vi "Process.vi"(8 "error in":errorcluster, 11 "DAQ_Manager":refnum<class "DAQ_Manager.lvclass">) -> (0 "error out":errorcluster, 3 "DAQ_Manager out":refnum<class "DAQ_Manager.lvclass">)   [LabVIEW 2016, in "DAQ_Manager.lvclass"]
doc: "---------------------------------------------------------------\nJKI State Machine Objects™\nhttp://jki.net/state-machine-objects/\nCopyright (C) 2005-2015, JKI <info@jki.net>\nALL RIGHTS RESERVED"
uses:
  DAQ_Manager.lvclass
  C:/Program Files (x86)/National Instruments/LabVIEW 2016/vi.lib/JKI/JKI SMO/SMO/SMO.lvclass
  DAQ/Typedefs/DAQ_Config.ctl
  DAQ/Typedefs/PrivateEvents--DAQ.AI.Channels.ctl
  DAQ/Typedefs/DAQ_Type.ctl
  DAQ/Typedefs/DAQ_SamplingInfo.ctl
  DAQ/Typedefs/DAQ_SamplingMode.ctl
  DAQmx.AI/Typedefs/DAQmx.AI_Config.ctl
  DAQmx.AI/Typedefs/AI.Coupling-enum.ctl
  DAQmx.AI/Typedefs/AI.Terminal-enum.ctl
  DAQmx.AO/Typedefs/DAQmx.AO_Config.ctl
  DAQmx.AO/Typedefs/AO.Terminal-enum.ctl
  <vilib>/JKI/JKI SMO/SMO/Typedefs/SMOState --Enum.ctl
  <vilib>/JKI/JKI SMO/SMO/Typedefs/Parent Call--Enum.ctl
  Typedefs/PrivateEvents--DAQ_Manager.setDAQConfig.ctl
  DAQ/Typedefs/PublicEvents--DAQ.Read.ctl
  DAQ/Typedefs/PublicEvents--DAQ.Write.ctl
  DAQ_Manager.lvclass/DAQ_Manager.ctl
  DAQ/DAQ.lvclass
  DAQmx/DAQmx.lvclass
  C:/user/patrick/hg/levy_inst_lockin.SMO/lvsrc/SMOs/DAQ/DAQ.lvclass
  DAQmx.AI/DAQmx.AI.lvclass
  C:/user/patrick/hg/levy_inst_lockin.SMO/lvsrc/SMOs/DAQmx/DAQmx.lvclass
  DAQmx.AO/DAQmx.AO.lvclass
  <vilib>/JKI/JKI SMO/SMO/SMO.lvclass
panel:
  out "Array":T1[](array[typedef])
  in  "Update Config?":bool
  in  "DAQmx.AO.config":T2[](array[typedef])=[{"output terminal configuration"=-1}] {"output terminal configuration" items=["Default"=-1, "RSE"=10083, "Differential"=10106, "Pseudodifferential"=12529]}
  in  "DAQmx.AI.config":T4[](array[typedef])=[{"AI.Coupling"=10045, "input terminal configuration "=-1}] {"input terminal configuration" items=["default"=-1, "RSE"=10083, "NRSE"=10078, "Differential"=10106, "Pseudodifferential"=12529]; "AI.Coupling" items=["AC"=10045, "DC"=10050, "GND"=10066]}
  in  "DAQ.Config (AO)":T7[](array[typedef])=[{"Channels"="PXI1Slot2/ao0", "DAQ_Type"=enum."AO", "minimum value"=-10.0, "maximum value"=10.0, "DAQ_SamplingInfo"={"Fs"=1000.0, "#s"=1000}, "DAQ_SamplingMode"=enum."Continuous"}] {"maximum value" format="%0.2f"; "minimum value" format="%0.2f"}
  in  "DAQ.Config (AI)":T7[](array[typedef])=[{"Channels"="PXI1Slot2/ai0", "DAQ_Type"=enum."AI", "minimum value"=-10.0, "maximum value"=10.0, "DAQ_SamplingInfo"={"Fs"=1000.0, "#s"=1000}, "DAQ_SamplingMode"=enum."Continuous"}] {"maximum value" format="%0.2f"; "minimum value" format="%0.2f"}
  in  "DAQmx Physical Channels (AO)":tag="PXI1Slot2/ao0:1, PXI1Slot3/ao0:1, PXI1Slot4/ao0:1, PXI1Slot5/ao0:1"
  in  "DAQmx Physical Channels (AI)":tag="PXI1Slot2/ai0:1, PXI1Slot3/ai0:1, PXI1Slot4/ai0:1, PXI1Slot5/ai0:1"
  in  "Simulate?":bool
  # "1. Make a lot of these controls hidden on default Main UI\n    (eg, output terminal)\n2. DAQ.Config etc should be arrays, with each element per device\n3. Make use of most recent lockin controls on front panel\n-- use new enums and arrays per channel/device\n4. DAQ_Manager needs an API for setting the DAQ config (setConfig?)\n5. In process.vi if any Config settings are changed: go to:\nDAQ: stop SMO\nDAQ: init\nDAQ: start SMO\n6. I don't think these need to be controls here in process.vi, they can just be\nchanged through public methods."
  # "DAQ Manager Process.vi"
  # "For instructions on how to use the JKI State Machine Objects, examples and video tutorials, visit:\nhttp://jki.net/state-machine-objects/\n\nJKI State Machine Objects™\nhttp://jki.net/state-machine-objects/\nCopyright (C) 2005-2015, JKI <info@jki.net>\nALL RIGHTS RESERVED"
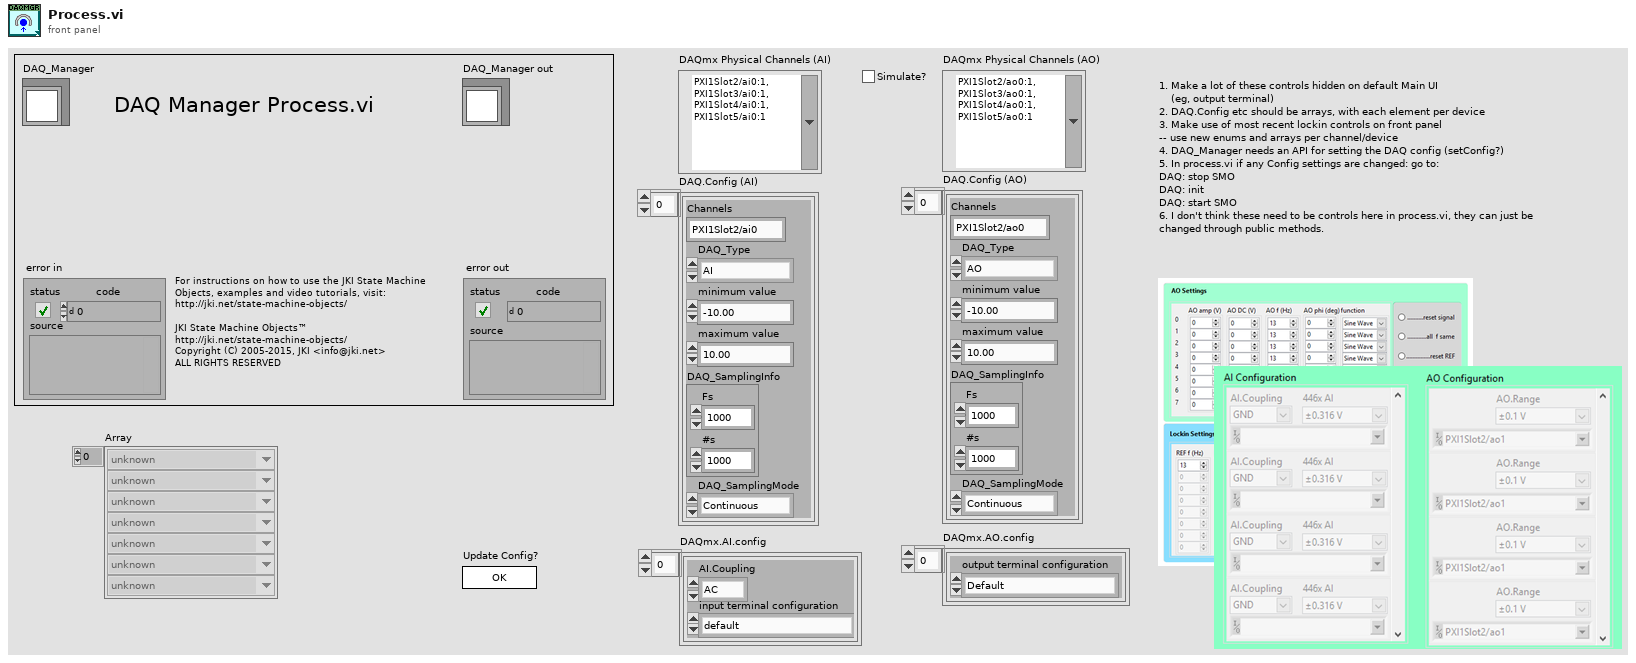
[diagram p1: front panel]
types:
  T1 = typedef "SMO.lvclass/SMOState --Enum.ctl" = enum16{"unknown", "Created", "Started", "Stopped"}
  T2 = typedef "DAQmx.AO.lvclass/DAQmx.AO_Config.ctl" = cluster{"output terminal configuration":T3}
  T3 = typedef "DAQmx.AO.lvclass/AO.Terminal-enum.ctl" = i32
  T4 = typedef "DAQmx.AI.lvclass/DAQmx.AI_Config.ctl" = cluster{"AI.Coupling":T5, "input terminal configuration ":T6}
  T5 = typedef "DAQmx.AI.lvclass/AI.Coupling-enum.ctl" = i32
  T6 = typedef "DAQmx.AI.lvclass/AI.Terminal-enum.ctl" = i32
  T7 = typedef "DAQ.lvclass/DAQ_Config.ctl" = cluster{"Channels":T8, "DAQ_Type":T9, "minimum value":dbl, "maximum value":dbl, "DAQ_SamplingInfo":T10, "DAQ_SamplingMode":T11}
  T8 = typedef "DAQ.lvclass/PrivateEvents--DAQ.AI.Channels.ctl" = string
  T9 = typedef "DAQ.lvclass/DAQ_Type.ctl" = enum16{"AI", "AO"}
  T10 = typedef "DAQ.lvclass/DAQ_SamplingInfo.ctl" = cluster{"Fs":dbl, "#s":i32}
  T11 = typedef "DAQ.lvclass/DAQ_SamplingMode.ctl" = enum16{"Continuous", "Finite"}
  T12 = typedef "SMO.lvclass/Parent Call--Enum.ctl" = enum16{"Allows parent to run", "Does not request parent to run"}
  T13 = typedef "DAQ_Manager.lvclass/PrivateEvents--DAQ_Manager.setDAQConfig.ctl" = cluster{"DAQ.Config (AI)":cluster{"Channels":string, "DAQ_Type":enum16{"AI", "AO"}, "minimum value":dbl, "maximum value":dbl, "DAQ_SamplingInfo":cluster{"Fs":dbl, "#s":i32}, "DAQ_SamplingMode":enum16{"Continuous", "Finite"}}[], "DAQmx.AI.config":T4[], "DAQ.Config (AO)":cluster{"Channels":string, "DAQ_Type":enum16{"AI", "AO"}, "minimum value":dbl, "maximum value":dbl, "DAQ_SamplingInfo":cluster{"Fs":dbl, "#s":i32}, "DAQ_SamplingMode":enum16{"Continuous", "Finite"}}[], "DAQmx.AO.config":T2[]}
  T14 = enum32{"invalid app kind", "Development System", "Run Time System", "Student Edition", "Embedded LabVIEW", "Evaluation", "Custom"}
  T15 = enum32{"Invalid", "Standard", "Closed", "Hidden", "Minimized", "Maximized"}
  T16 = enum32{"Bad", "Idle", "Run top level", "Running"}
  T17 = typedef "DAQ.lvclass/PublicEvents--DAQ.Read.ctl" = waveform(dbl)[]
  T18 = cluster{"Core":cluster{"Current VI Reference":refnum<vi>, "Close Panel on Exit?":bool, "error":errorcluster}, "Self Reference":refnum<class "DAQ_Manager.lvclass">, "Your string data":string, "DAQ":refnum<class "DAQ.lvclass">[], "setWaveform":T17, "to":i32, "AI events":refnum<user-event>[], "DAQ.Config (AO)":T7[], "DAQ.Config (AI)":T7[], "DAQmx.AO.Config":T2[], "DAQmx.AI.Config":T4[]}
  T19 = cluster{"Channels":string, "DAQ_Type":enum16{"AI", "AO"}, "minimum value":dbl, "maximum value":dbl, "DAQ_SamplingInfo":cluster{"Fs":dbl, "#s":i32}, "DAQ_SamplingMode":enum16{"Continuous", "Finite"}}[]
  T20 = typedef "DAQ_Manager.lvclass/PrivateEvents--DAQ_Manager.setWaveform.ctl" = waveform(dbl)[]
  T21 = cluster{"Current VI Reference":refnum<vi>, "Close Panel on Exit?":bool, "error":errorcluster}
  T22 = typedef "SMO.lvclass/Protected Events.ctl" = cluster{"StopProcesses":refnum<user-event>, "AbortProcesses":refnum<user-event>, "Config Changed":refnum<user-event>, "Dependency":refnum<user-event>}
  T23 = typedef "DAQ_Manager.lvclass/PrivateEvents--Cluster.ctl" = cluster{"setWaveform":refnum<user-event>, "setDAQConfig":refnum<user-event>}
  T24 = typedef "DAQ_Manager.lvclass/PublicEvents--Cluster.ctl" = cluster{"getWaveform":refnum<user-event>}
  T25 = typedef "DAQ.lvclass/PublicEvents--Cluster.ctl" = cluster{"DAQ.Read":refnum<user-event>, "DAQ.Write":refnum<user-event>}
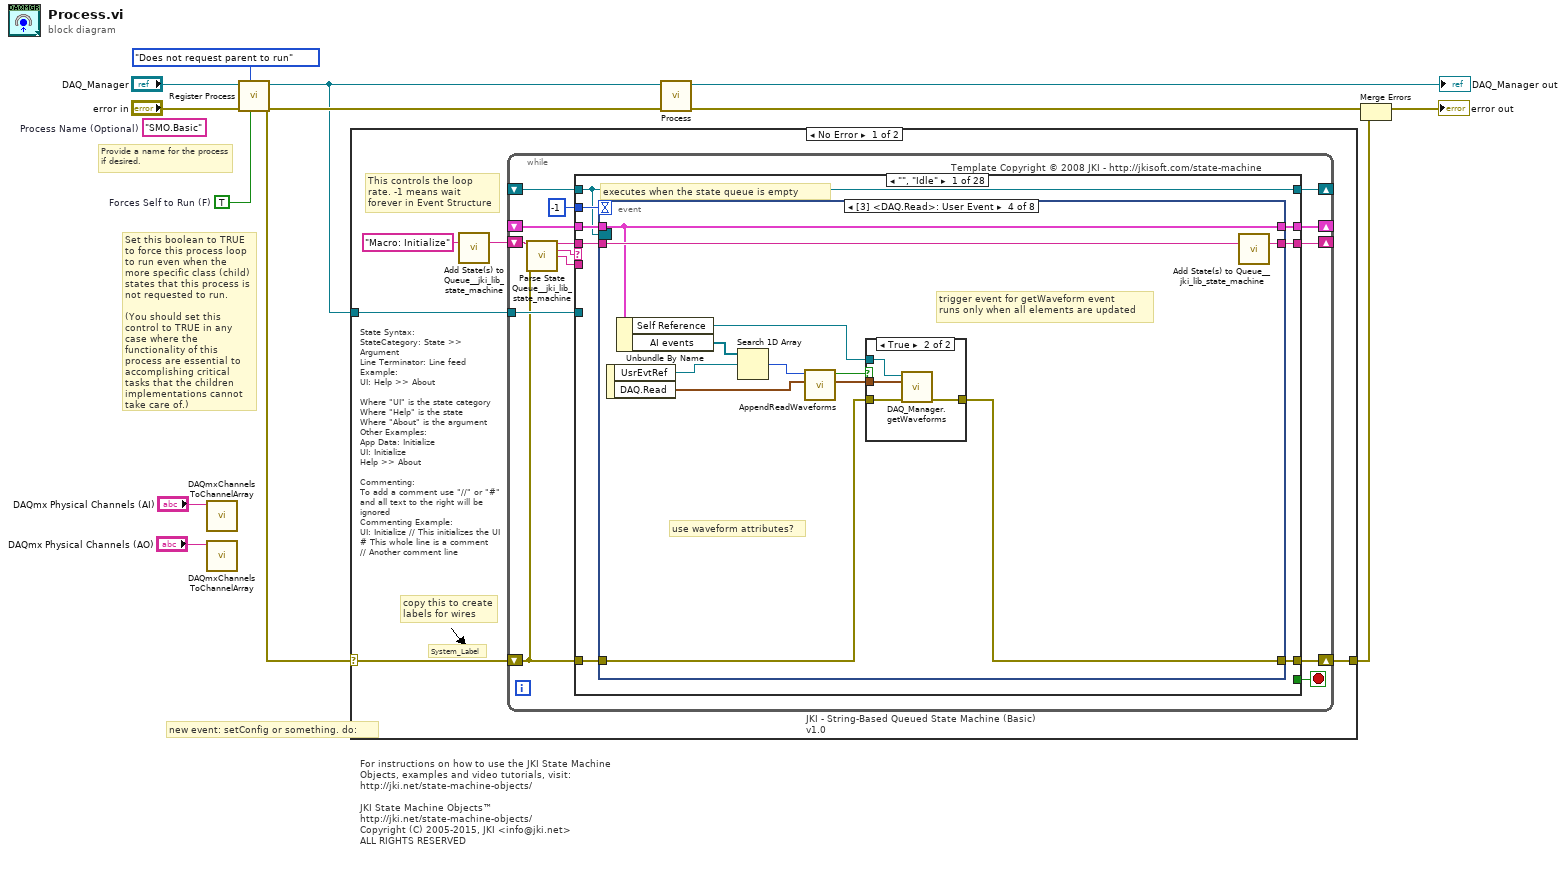
[diagram p0: block diagram]
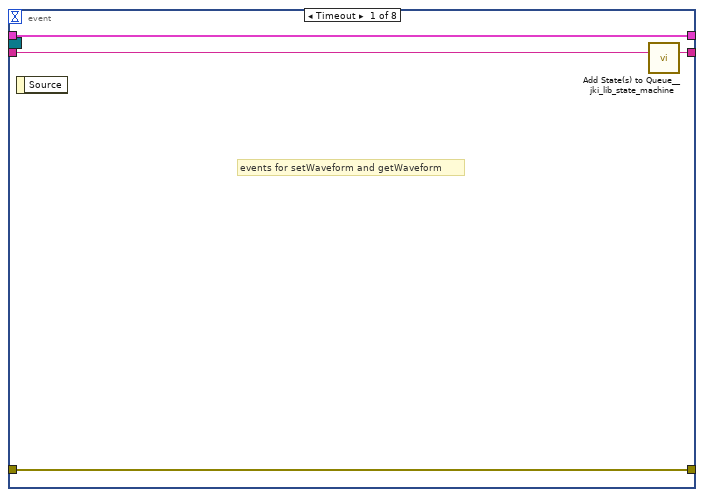
[diagram p2: hidden frame]
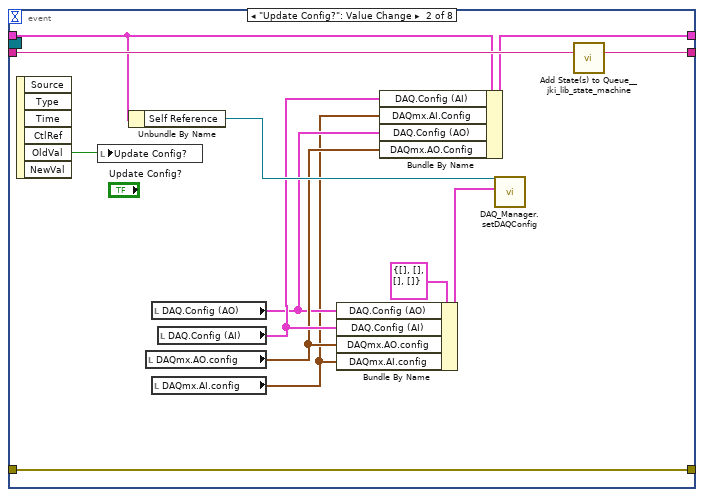
[diagram p3: hidden frame]
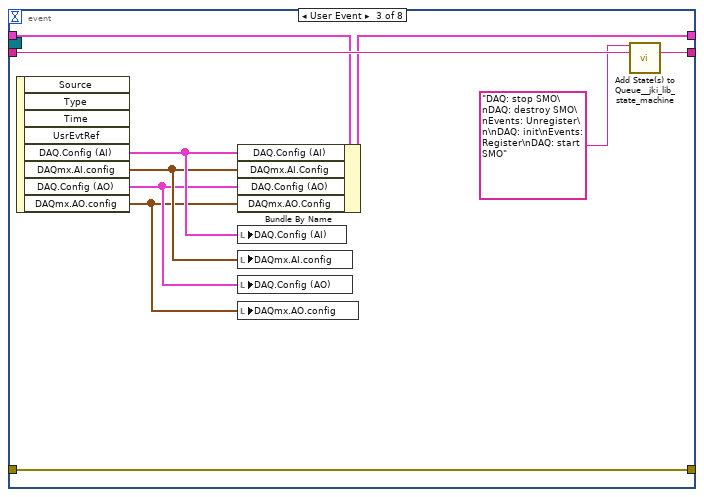
[diagram p4: hidden frame]
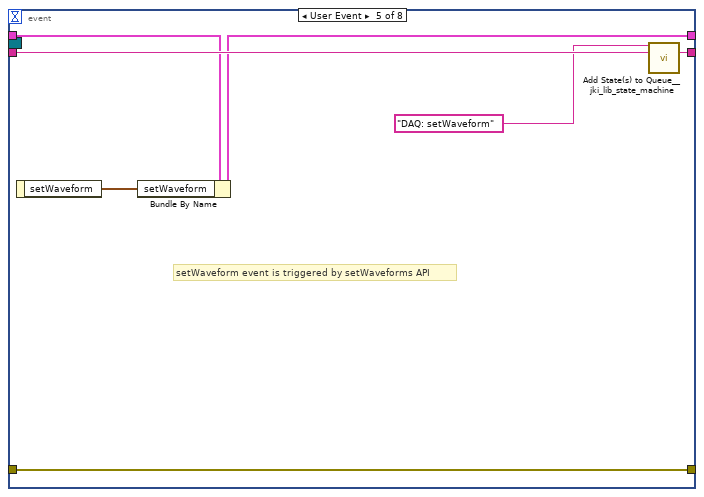
[diagram p6: hidden frame]
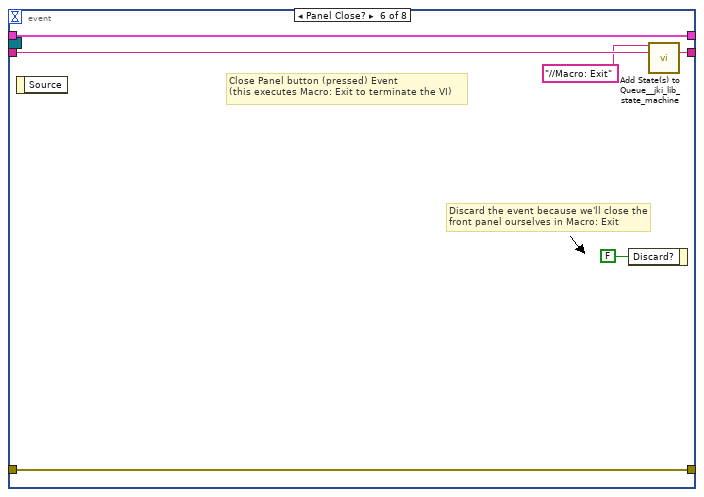
[diagram p7: hidden frame]
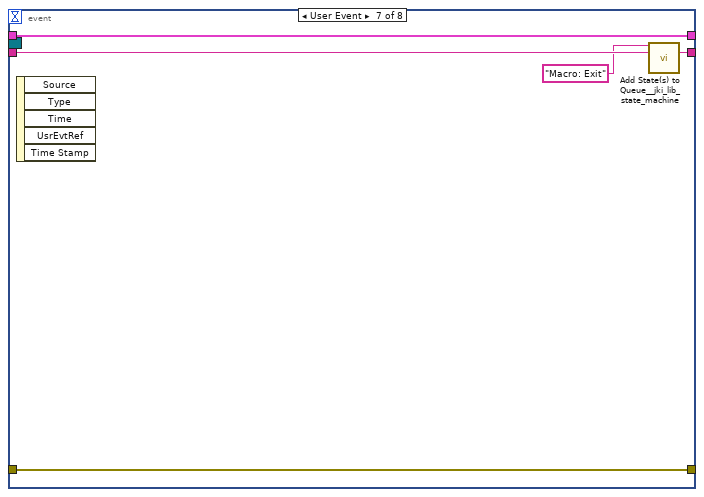
[diagram p8: hidden frame]
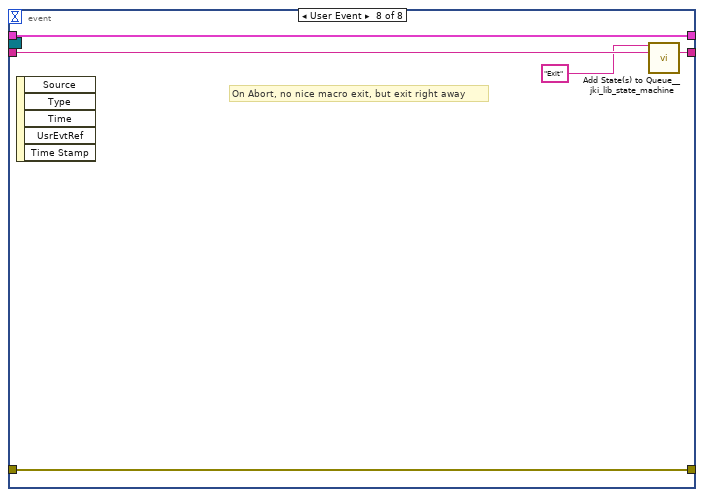
[diagram p9: hidden frame]
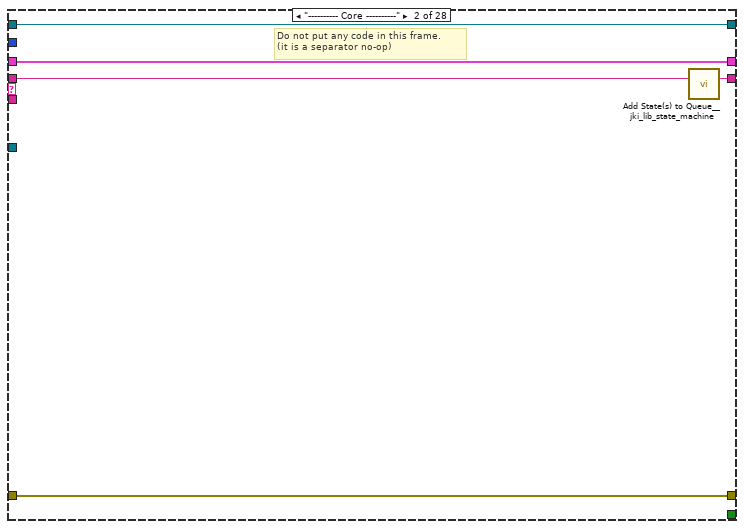
[diagram p10: hidden frame]
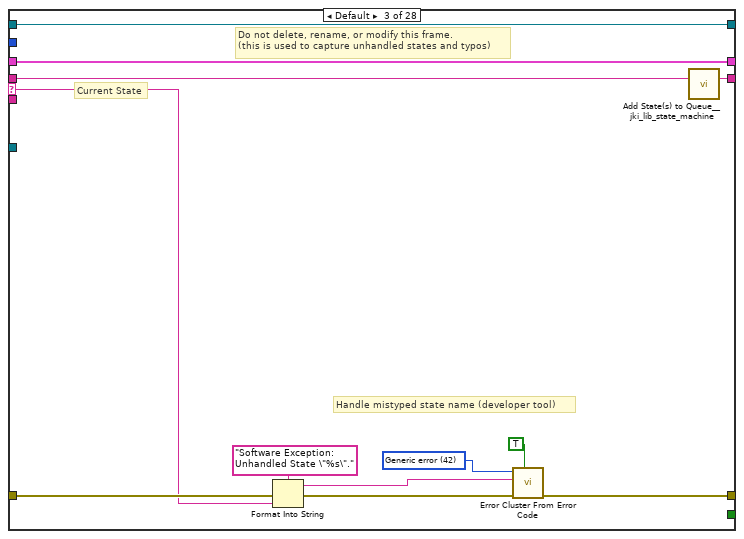
[diagram p11: hidden frame]
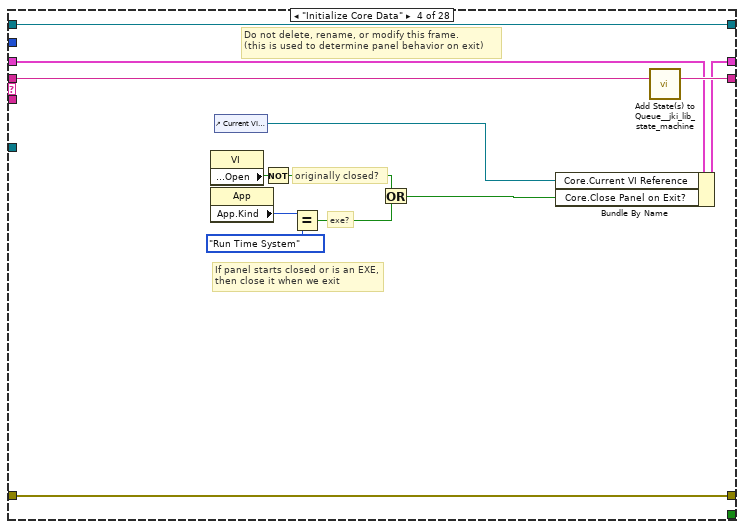
[diagram p12: hidden frame]
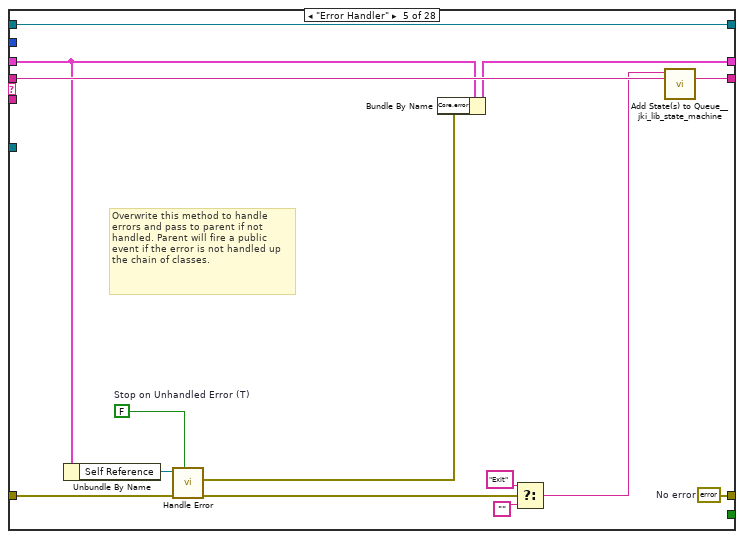
[diagram p13: hidden frame]
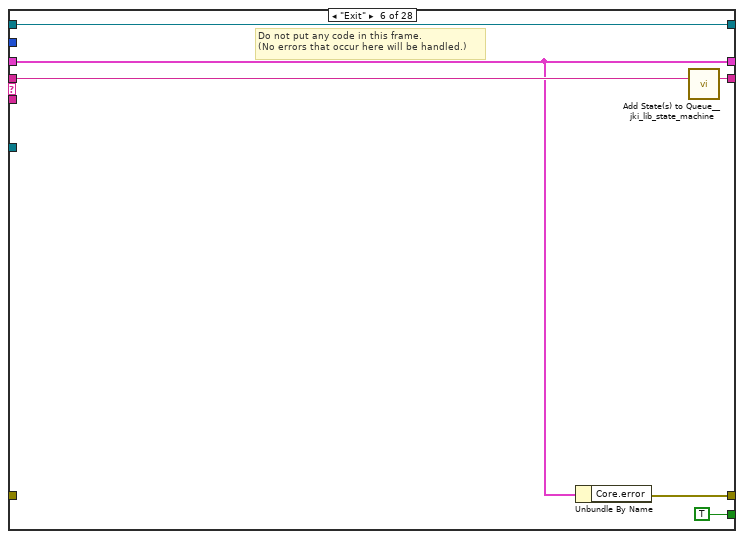
[diagram p14: hidden frame]
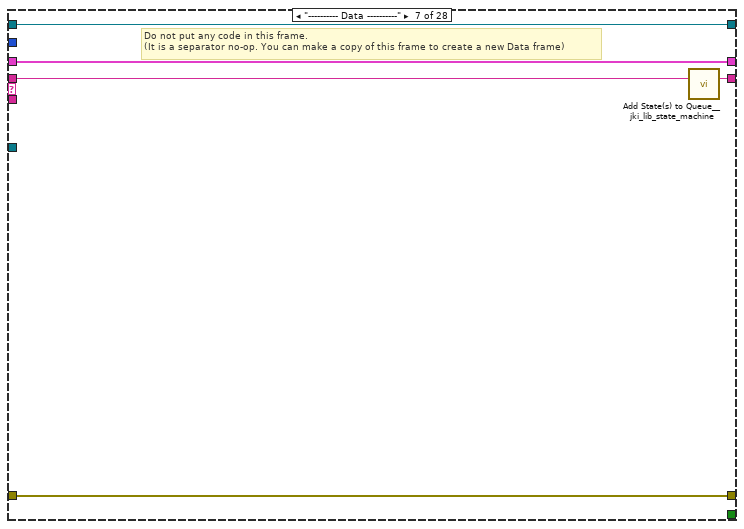
[diagram p15: hidden frame]
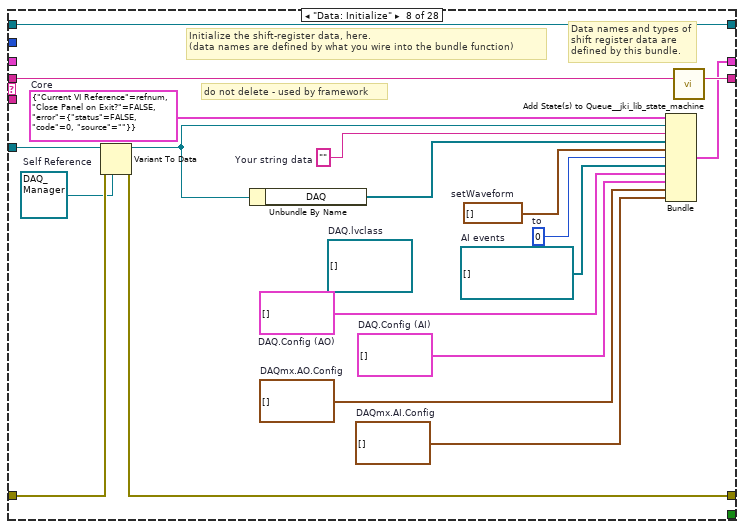
[diagram p16: hidden frame]
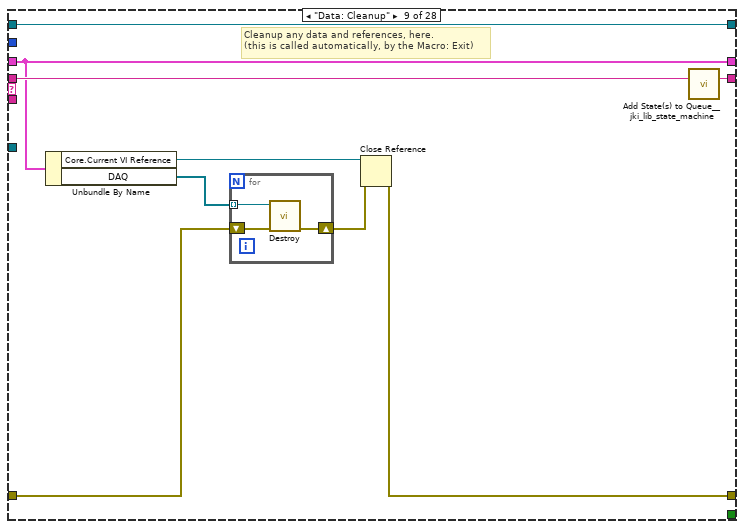
[diagram p17: hidden frame]
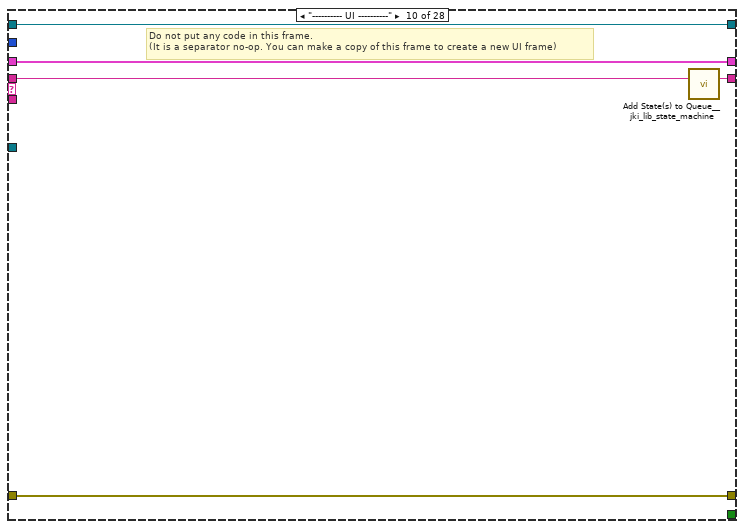
[diagram p18: hidden frame]
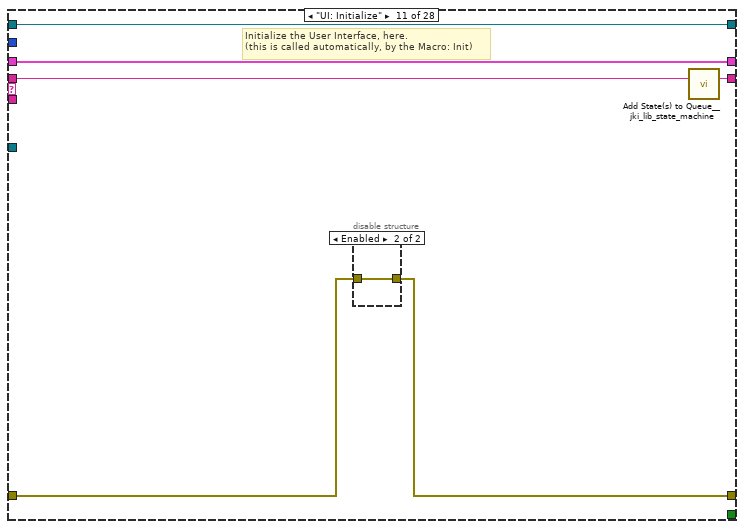
[diagram p19: hidden frame]
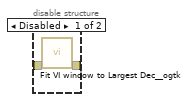
[diagram p20: hidden frame]
diagram:
  w3 = TRUE  # Forces Self to Run (F)
  (unwired) "SMO.Basic"  # Process Name (Optional)
  # "new event: setConfig or something. do:"
  # "Provide a name for the process\nif desired."
  # "Set this boolean to TRUE to force this process loop to run even when the more specific class (child) states that this process is not requested to run.\n\n(You should set this control to TRUE in any case where the functionality of this process are essential to accomplishing critical tasks that the children implementations cannot take care of.)"
  # "For instructions on how to use the JKI State Machine Objects, examples and video tutorials, visit:\nhttp://jki.net/state-machine-objects/\n\nJKI State Machine Objects™\nhttp://jki.net/state-machine-objects/\nCopyright (C) 2005-2015, JKI <info@jki.net>\nALL RIGHTS RESERVED"
  n1 = call "DAQmxChannelsToChannelArray.vi"("DAQmx Physical Channel"="DAQmx Physical Channels (AI)") -> ()  [unwired: 10 in, 1 out]
  n2 = call "DAQmxChannelsToChannelArray.vi"("DAQmx Physical Channel"="DAQmx Physical Channels (AO)") -> ()  [unwired: 10 in, 1 out]
  n3 = call <vilib>:"Register Process.vi"("Forces Self to Run (F)"=w3, "Parent Call"=Parent_Call--Enum."Does not request parent to run", "error in (no error)"="error in", "SMO"="DAQ_Manager") -> ("error out"=w9:errorcluster, "SMO out"=w8:refnum<class "DAQ_Manager.lvclass">)  [unwired: 6 in]
  n4 = case shown="No Error" w9 {
    selector: w9 -> [w14 w461]
    tunnel: w8 -> [w15 _]
    tunnel: [w13 w461] -> w5
    frame No Error {
      # "State Syntax:\nStateCategory: State >> Argument\nLine Terminator: Line feed\nExample:\nUI: Help >> About\n\nWhere \"UI\" is the state category\nWhere \"Help\" is the state\nWhere \"About\" is the argument\nOther Examples:\nApp Data: Initialize\nUI: Initialize\nHelp >> About\n\nCommenting:\nTo add a comment use \"//\" or \"#\" and all text to the right will be ignored\nCommenting Example:\nUI: Initialize // This initializes the UI\n# This whole line is a comment\n// Another comment line"
      # "copy this to create labels for wires"
      # "This controls the loop rate. -1 means wait forever in Event Structure"
      # "System_Label"
      n5 = call <vilib>:"Add State(s) to Queue__jki_lib_state_machine.vi"("State(s) in (\"\")"="Macro: Initialize") -> ("States Out"=w17:string)  [unwired: 14 in]
      n6 = while "JKI - String-Based Queued State Machine (Basic) v1.0" {
        shift-right: [w25] -> _
        shift-left: _ -> [w20]
        shift-right: [w19] -> w13
        shift-left: w14 -> [w21]
        shift-right: [w27] -> _
        shift-left: w17 -> [w28]
        tunnel: w15 -> [w24]
        shift-right: [w23] -> _
        shift-left: _ -> [w22]
        stop <- w26 stop-if-true
        # "Template Copyright © 2008 JKI - http://jkisoft.com/state-machine"
        n7 = call <vilib>:"Parse State Queue__jki_lib_state_machine.vi"("State Queue"=w28, "Error In (no error)"=w21) -> ("Remaining States"=w30:string, "Current State"=w31:string, "Arguments"=w29:string)  [unwired: 11 in]
        n8 = case shown="\"\", \"Idle\"" w31 {
          selector: w31 -> [_ _ w113 _ _ _ _ _ _ _ _ _ _ _ _ _ _ _ _ _ _ _ _ _ _ _ _ _]
          tunnel: w30 -> [w39 w111 w117 w136 w150 w156 w161 w180 w189 w197 w203 w213 w231 w263 w277 w292 w297 w308 w313 w332 w343 w348 w363 w411 w423 w437 w449 w460]
          tunnel: w29 -> [_ _ _ _ _ _ _ _ _ _ _ w207 w226 _ _ _ _ _ _ _ _ _ _ _ _ _ _ _]
          tunnel: w20 -> [w37 w108 w115 w127 w144 w152 w158 _ w185 w194 w200 w211 w228 w260 w273 w283 w294 w305 w310 w323 w341 w346 w352 w404 w420 w434 w442 w457]
          tunnel: [w38 w110 w116 w135 w149 w155 w160 w179 w188 w196 w202 w212 w230 w262 w276 w291 w296 w307 w312 w331 w342 w347 w362 w410 w422 w436 w448 w459] -> w27
          tunnel: [_ _ _ _ _ TRUE _ _ _ _ _ _ _ _ _ _ _ _ _ _ _ _ _ _ _ _ _ _] -> w26
          tunnel: [w34 w108 w115 w134 w143 w152 w158 w170 w185 w194 w200 w211 w228 w260 w273 w283 w294 w305 w310 w322 w341 w346 w360 w404 w420 w434 w441 w457] -> w25
          tunnel: -1 ("to") -> [w33 _ _ _ _ _ _ _ _ _ _ _ _ _ _ _ _ _ _ _ _ _ _ _ _ _ _ _]
          tunnel: w24 -> [_ _ _ _ _ _ _ w174 _ _ _ _ _ _ _ _ _ _ _ _ _ _ _ _ _ _ _ _]
          tunnel: [w32 w107 w112 w124 w148 w153 w157 w173 w184 w193 w201 w210 w225 w259 w274 w284 w293 w306 w309 w330 w340 w345 w361 w409 w421 w435 w450 w458] -> w23
          tunnel: w22 -> [w32 w107 w112 w124 w148 w153 w157 w173 w184 w193 w201 w210 w225 w259 w274 w284 w293 w306 w309 _ w340 w345 w361 w409 w421 w435 w450 w458]
          tunnel: w21 -> [w35 w109 w118 w133 w146 _ w159 w177 w183 w195 w199 w209 w229 w261 w275 w290 w295 w300 w311 w327 w339 w344 w353 w408 w419 w433 w447 w453]
          tunnel: [w36 w109 w119 w133 w145 w151 w159 w176 w186 w195 w198 w208 w223 w261 w275 w290 w295 w299 w311 w328 w339 w344 w354 w407 w417 w431 w447 w454] -> w19
          frame "", "Idle" {
            # "executes when the state queue is empty"
            n9 = event shown="[3] <DAQ.Read>: User Event" {
              selector: w32 -> [_ _ _ _ _ _ _ _]
              dyn-events: _ -> [_ _ _ _ _ _ _ _]
              timeout: w33 -> [_ _ _ _ _ _ _ _]
              tunnel: w39 -> [w43 w55 w65 w78 w90 w96 w101 w106]
              tunnel: [w42 w56 w66 w77 w89 w95 w100 w105] -> w38
              tunnel: w37 -> [w41 w49 w62 w76 w86 w93 w98 w103]
              tunnel: [w40 w53 w63 w69 w88 w94 w99 w104] -> w36
              tunnel: w35 -> [w40 w53 w63 w70 w88 w94 w99 w104]
              tunnel: [w41 w48 w61 w76 w85 w93 w98 w103] -> w34
              event Timeout {
                # "events for setWaveform and getWaveform"
                n10 = event-data() -> ()  [unwired: 1 in, 1 out]
                n11 = call <vilib>:"Add State(s) to Queue__jki_lib_state_machine.vi"("State(s) in (\"\")"=w43) -> ("States Out"=w42:string)  [unwired: 14 in]
              }
              event "Update Config?": Value Change {
                n12 = event-data() -> ("OldVal"=w54:bool)  [unwired: 1 in, 5 out]
                n13 = local write "Update Config?"(w54) -> ()
                n14 = Unbundle By Name(w49) -> ("Self Reference"=w50:refnum<class "DAQ_Manager.lvclass">)
                n15 = local read "DAQmx.AO.config"() -> (w46:T2[])
                n16 = local read "DAQ.Config (AO)"() -> (w45:T7[])
                n17 = local read "DAQmx.AI.config"() -> (w44:T4[])
                n18 = local read "DAQ.Config (AI)"() -> (w47:T7[])
                n19 = Bundle By Name(cluster=T13 {"DAQ.Config (AI)"=[], "DAQmx.AI.config"=[], "DAQ.Config (AO)"=[], "DAQmx.AO.config"=[]} ("DAQ_Manager.setDAQConfig"), "DAQ.Config (AO)"=w45, "DAQ.Config (AI)"=w47, "DAQmx.AO.config"=w46, "DAQmx.AI.config"=w44) -> (w51:T13)
                n20 = Bundle By Name(cluster=w49, "DAQ.Config (AI)"=w47, "DAQmx.AI.Config"=w44, "DAQ.Config (AO)"=w45, "DAQmx.AO.Config"=w46) -> (w48:T18)
                n21 = call "DAQ_Manager.setDAQConfig.vi"("DAQ_Manager.setDAQConfig"=w51, "DAQ_Manager"=w50) -> ()  [unwired: 8 in, 2 out]
                n22 = call <vilib>:"Add State(s) to Queue__jki_lib_state_machine.vi"("State(s) in (\"\")"=w55) -> ("States Out"=w56:string)  [unwired: 14 in]
              }
              event User Event {
                n23 = event-data() -> ("DAQ.Config (AI)"=w60:T19, "DAQmx.AI.config"=w59:T4[], "DAQ.Config (AO)"=w58:T19, "DAQmx.AO.config"=w57:T2[])  [unwired: 1 in, 4 out]
                n24 = Bundle By Name(cluster=w62, "DAQ.Config (AI)"=w60, "DAQmx.AI.Config"=w59, "DAQ.Config (AO)"=w58, "DAQmx.AO.Config"=w57) -> (w61:T18)
                n25 = local write "DAQ.Config (AI)"(w60) -> ()
                n26 = local write "DAQmx.AI.config"(w59) -> ()
                n27 = local write "DAQ.Config (AO)"(w58) -> ()
                n28 = local write "DAQmx.AO.config"(w57) -> ()
                n29 = call <vilib>:"Add State(s) to Queue__jki_lib_state_machine.vi"("State(s) in Front (\"\")"="DAQ: stop SMO\nDAQ: destroy SMO\nEvents: Unregister\n\nDAQ: init\nEvents: Register\nDAQ: start SMO" ("State(s) in Front (\"\")"), "State(s) in (\"\")"=w65) -> ("States Out"=w66:string)  [unwired: 13 in]
              }
              event User Event {
                # "use waveform attributes?"
                # "trigger event for getWaveform event\nruns only when all elements are updated"
                n30 = event-data() -> ("UsrEvtRef"=w74:refnum<user-event>, "DAQ.Read"=w67:waveform(dbl)[])  [unwired: 1 in]
                n31 = Unbundle By Name(w76) -> ("Self Reference"=w71:refnum<class "DAQ_Manager.lvclass">, "AI events"=w75:refnum<user-event>[])
                n32 = Search 1D Array(1D array=w75, element=w74) -> (index of element=w68:i32)  [unwired: 1 in]
                n33 = call "AppendReadWaveforms.vi"("WFM in"=w67, "index of element"=w68) -> ("WFM out"=w73:waveform(dbl)[], "x = y?"=w72:bool)  [unwired: 8 in]
                n34 = case shown="True" w72 {
                  tunnel: w73 -> [_ w83]
                  tunnel: w71 -> [_ w82]
                  tunnel: w70 -> [w79 w81]
                  tunnel: [w79 w80] -> w69
                  frame False {
                  }
                  frame True {
                    n35 = call "DAQ_Manager.getWaveforms.vi"("error in (no error)"=w81, "getWaveform"=w83, "DAQ_Manager"=w82) -> ("error out"=w80:errorcluster)  [unwired: 7 in, 1 out]
                  }
                }
                n36 = call <vilib>:"Add State(s) to Queue__jki_lib_state_machine.vi"("State(s) in (\"\")"=w78) -> ("States Out"=w77:string)  [unwired: 14 in]
              }
              event User Event {
                # "setWaveform event is triggered by setWaveforms API"
                n37 = event-data() -> ("setWaveform"=w87:T20)  [unwired: 1 in]
                n38 = Bundle By Name(cluster=w86, "setWaveform"=w87) -> (w85:T18)
                n39 = call <vilib>:"Add State(s) to Queue__jki_lib_state_machine.vi"("State(s) in Front (\"\")"="DAQ: setWaveform" ("State(s) in Front (\"\")"), "State(s) in (\"\")"=w90) -> ("States Out"=w89:string)  [unwired: 13 in]
              }
              event Panel Close? {
                # "Discard the event because we'll close the front panel ourselves in Macro: Exit"
                # "Close Panel button (pressed) Event\n(this executes Macro: Exit to terminate the VI)"
                n40 = event-data() -> ()  [unwired: 1 in, 1 out]
                n41 = event-data("Discard?"=FALSE) -> ()  [unwired: 1 in, 1 out]
                n42 = call <vilib>:"Add State(s) to Queue__jki_lib_state_machine.vi"("State(s) in Front (\"\")"="//Macro: Exit", "State(s) in (\"\")"=w96) -> ("States Out"=w95:string)  [unwired: 13 in]
              }
              event User Event {
                n43 = event-data() -> ()  [unwired: 1 in, 5 out]
                n44 = call <vilib>:"Add State(s) to Queue__jki_lib_state_machine.vi"("State(s) in Front (\"\")"="Macro: Exit", "State(s) in (\"\")"=w101) -> ("States Out"=w100:string)  [unwired: 13 in]
              }
              event User Event {
                # "On Abort, no nice macro exit, but exit right away"
                n45 = event-data() -> ()  [unwired: 1 in, 5 out]
                n46 = call <vilib>:"Add State(s) to Queue__jki_lib_state_machine.vi"("State(s) in Front (\"\")"="Exit", "State(s) in (\"\")"=w106) -> ("States Out"=w105:string)  [unwired: 13 in]
              }
            }
          }
          frame "---------- Core ----------" {
            # "Do not put any code in this frame.\n(it is a separator no-op)"
            n47 = call <vilib>:"Add State(s) to Queue__jki_lib_state_machine.vi"("State(s) in (\"\")"=w111) -> ("States Out"=w110:string)  [unwired: 14 in]
          }
          frame Default {
            w122 = 42 items=["No error", "Argument error", "Memory is full", "Out of zone", "End of file", "File already open", "Generic file I/O error", "File not found", "File permission error", "Disk is full", "Duplicate path", "Too many files open", "System feature not enabled", "Resource file not found", "Cannot add resource", "Resource not found", "Image not found", "Image memory error", "Pen does not exist", "Config type invalid", "Config token not found", "Config parse error", "Config memory error", "Bad external code format", "Bad external code offset", "External code not present", "Null window", "Destroy window error", "Null menu", "Print aborted", "Bad print record", "Print driver error", "Windows error during printing", "Memory error during printing", "Print dialog error", "Generic print error", "Invalid device refnum", "Device not found", "Device parameter error", "Device unit error", "Cannot open device", "Device call aborted", "Generic error", "Cancelled by user", "Object ID too low", "Object ID too high", "Object not in heap", "Unknown heap", "Unknown object (invalid DefProc)", "Unknown object (DefProc not in table)", "Message out of range", "Invalid (null) method", "Unknown message", "Manager call not supported", "Bad address", "Network operation in progress", "Network operation timed out", "Connection is busy", "Network attribute not supported", "Network error", "Address in use", "System out of memory", "Connection aborted", "Connection refused", "Not connected", "Already connected", "Connection closed", "Initialization error (interapplication manager)", "Bad occurrence", "Wait on unbound occurrence handler", "Occurrence queue overflow", "Datalog type conflict", "Unused", "Unrecognized type (interapplication manager)", "Memory corrupt", "Failed to make temporary DLL", "Old CIN version", "Drag socket not found", "Failed to load drop-object", "Failed to register OLE object", "Failed to release OLE object", "Format specifier type mismatch", "Unknown format specifier", "Too few format specifiers", "Too many format specifiers", "Scan failed", "Newer CIN version", "Error converting to variant", "Runtime menu error", "Password tampered", "Variant attribute not found", "Incompatible variant data type", "Event data is not available", "Event Store is not present", "Occurrence is not found", "Event Queue is not created", "Event info is not available", "Refnum passed is NULL", "Error retrieving Class GUID", "Error retrieving CoClass GUID", "Error retrieving TypeLib GUID.", "Bad built application magic bytes.", "Specific driver is different from the specific driver associated with the Logical Name.", "There is no session opened to the class driver.", "Max Error", "MAX - Error with config objects", "MAX - Error loading configuration", "MAX - Group not supported"]
            # "Current State"
            # "Do not delete, rename, or modify this frame.\n(this is used to capture unhandled states and typos)"
            # "Handle mistyped state name (developer tool)"
            n48 = Format Into String(format string="Software Exception: Unhandled State \"%s\"." ("message"), error in=w118, w113) -> (resulting string=w121:string, error out=w120:errorcluster)  [unwired: 1 in]
            n49 = call <vilib>:"Error Cluster From Error Code.vi"("show call chain? (False)"=TRUE, "error in (no error)"=w120, "error message (\"\")"=w121, "error code (0)"=w122) -> ("error out"=w119:errorcluster)  [unwired: 5 in]
            n50 = call <vilib>:"Add State(s) to Queue__jki_lib_state_machine.vi"("State(s) in (\"\")"=w117) -> ("States Out"=w116:string)  [unwired: 14 in]
          }
          frame "Initialize Core Data" {
            # "Do not delete, rename, or modify this frame.\n(this is used to determine panel behavior on exit)"
            # "originally closed?"
            # "exe?"
            # "If panel starts closed or is an EXE, then close it when we exit"
            n51 = property class="VI"() -> ("Front Panel.Open"=w132:bool)  [unwired: 2 in, 2 out]
            n52 = property class="App"() -> ("App.Kind"=w131:T14)  [unwired: 2 in, 2 out]
            n53 = control-ref of="Current VI Reference"() -> (w125:refnum<vi>)
            n54 = Not(x=w132) -> (.not. x?=w129:bool)
            n55 = Equal?(x=w131, y=T14."Run Time System" ("Application:Kind")) -> (x = y?=w128:bool)
            n56 = Or(x=w129, y=w128) -> (x .or. y?=w126:bool)
            n57 = Bundle By Name(cluster=w127, "Core.Current VI Reference"=w125, "Core.Close Panel on Exit?"=w126) -> (w134:T18)
            n58 = call <vilib>:"Add State(s) to Queue__jki_lib_state_machine.vi"("State(s) in (\"\")"=w136) -> ("States Out"=w135:string)  [unwired: 14 in]
          }
          frame "Error Handler" {
            w137 = FALSE  # Stop on Unhandled Error (T)
            w145 = errorcluster {"status"=FALSE, "code"=0, "source"=""}  # No error
            # "Overwrite this method to handle errors and pass to parent if not handled. Parent will fire a public event if the error is not handled up the chain of classes."
            n59 = Unbundle By Name(w144) -> ("Self Reference"=w147:refnum<class "DAQ_Manager.lvclass">)
            n60 = call-dynamic "Handle Error.vi"("Stop on Unhandled Error (T)"=w137, "error in"=w146, "SMO"=w147) -> ("handling error"=w138:errorcluster, "Unhandled error"=w141:errorcluster)  [unwired: 6 in, 1 out]
            n61 = Bundle By Name(cluster=w144, "Core.error"=w141) -> (w143:T18)
            n62 = Select(t="Exit", s=w138, f="") -> (s? t:f=w142:string)
            n63 = call <vilib>:"Add State(s) to Queue__jki_lib_state_machine.vi"("State(s) in Front (\"\")"=w142, "State(s) in (\"\")"=w150) -> ("States Out"=w149:string)  [unwired: 13 in]
          }
          frame "Exit" {
            # "Do not put any code in this frame.\n(No errors that occur here will be handled.)"
            n64 = Unbundle By Name(w152) -> ("Core.error"=w151:errorcluster)
            n65 = call <vilib>:"Add State(s) to Queue__jki_lib_state_machine.vi"("State(s) in (\"\")"=w156) -> ("States Out"=w155:string)  [unwired: 14 in]
          }
          frame "---------- Data ----------" {
            # "Do not put any code in this frame.\n(It is a separator no-op. You can make a copy of this frame to create a new Data frame)"
            n66 = call <vilib>:"Add State(s) to Queue__jki_lib_state_machine.vi"("State(s) in (\"\")"=w161) -> ("States Out"=w160:string)  [unwired: 14 in]
          }
          frame "Data: Initialize" {
            w164 = T4[] []  # DAQmx.AI.Config
            w165 = T2[] []  # DAQmx.AO.Config
            w166 = T7[] []  # DAQ.Config (AI)
            w167 = T7[] []  # DAQ.Config (AO)
            w168 = refnum<user-event>[] []  # AI events
            w169 = T17 []  # setWaveform
            w171 = 0  # to
            (unwired) refnum<class "DAQ.lvclass">[] []  # DAQ.lvclass
            w172 = T21 {"Current VI Reference"=refnum, "Close Panel on Exit?"=FALSE, "error"={"status"=FALSE, "code"=0, "source"=""}}  # Core
            w175 = refnum<class "DAQ_Manager.lvclass"> refnum  # Self Reference
            w178 = ""  # Your string data
            # "do not delete - used by framework"
            # "Data names and types of shift register data are defined by this bundle."
            # "Initialize the shift-register data, here.\n(data names are defined by what you wire into the bundle function)"
            n67 = Variant To Data(error in=w177, type=w175, Variant=w174) -> (data=w163:refnum<class "DAQ_Manager.lvclass">, error out=w176:errorcluster)
            n68 = Unbundle By Name(w163) -> ("DAQ"=w162:refnum<class "DAQ.lvclass">[])
            n69 = Bundle("Core"=w172, "Self Reference"=w163, "Your string data"=w178, "DAQ"=w162, "setWaveform"=w169, "to"=w171, "AI events"=w168, "DAQ.Config (AO)"=w167, "DAQ.Config (AI)"=w166, "DAQmx.AO.Config"=w165, "DAQmx.AI.Config"=w164) -> (w170:T18)  [unwired: 1 in]
            n70 = call <vilib>:"Add State(s) to Queue__jki_lib_state_machine.vi"("State(s) in (\"\")"=w180) -> ("States Out"=w179:string)  [unwired: 14 in]
          }
          frame "Data: Cleanup" {
            # "Cleanup any data and references, here.\n(this is called automatically, by the Macro: Exit)"
            n71 = Unbundle By Name(w185) -> ("Core.Current VI Reference"=w187:refnum<vi>, "DAQ"=w181:refnum<class "DAQ.lvclass">[])
            n72 = for {
              tunnel: w181 -> [w190] mode=indexing
              shift-right: [w192] -> w182
              shift-left: w183 -> [w191]
              n73 = call <vilib>:"Destroy.vi"("error in (no error)"=w191, "SMO"=w190) -> ("error out"=w192:errorcluster)  [unwired: 9 in]
            }
            n74 = Close Reference(reference=w187, error in (no error)=w182) -> (error out=w186:errorcluster)
            n75 = call <vilib>:"Add State(s) to Queue__jki_lib_state_machine.vi"("State(s) in (\"\")"=w189) -> ("States Out"=w188:string)  [unwired: 14 in]
          }
          frame "---------- UI ----------" {
            # "Do not put any code in this frame.\n(It is a separator no-op. You can make a copy of this frame to create a new UI frame)"
            n76 = call <vilib>:"Add State(s) to Queue__jki_lib_state_machine.vi"("State(s) in (\"\")"=w197) -> ("States Out"=w196:string)  [unwired: 14 in]
          }
          frame "UI: Initialize" {
            # "Initialize the User Interface, here.\n(this is called automatically, by the Macro: Init)"
            n77 = disable-structure shown="Enabled" {
              disable-tunnel: w199 -> [w205 w206]
              disable-tunnel: [w204 w206] -> w198
              frame Disabled {
                n78 = call <userlib>:"Fit VI window to Largest Dec__ogtk.vi"("error in (no error)"=w205) -> ("error out"=w204:errorcluster)  [unwired: 5 in, 1 out]
              }
              frame Enabled {
              }
            }
            n79 = call <vilib>:"Add State(s) to Queue__jki_lib_state_machine.vi"("State(s) in (\"\")"=w203) -> ("States Out"=w202:string)  [unwired: 14 in]
          }
          frame "UI: Cursor Set" {
            # "Argument"
            # "Initialize the User Interface, here.\n(this is called automatically, by the Macro: Init)"
            n80 = disable-structure shown="Default" {
              disable-tunnel: w209 -> [w214 w217]
              disable-tunnel: [w214 w216] -> w208
              disable-tunnel: w207 -> [_ w215]
              frame condition #0 {
              }
              frame condition #1 (active) {
                n81 = case shown="\"Idle\", Default" w215 {
                  tunnel: w217 -> [w219 w221]
                  tunnel: [w218 w220] -> w216
                  frame "Idle", Default {
                    n82 = call <vilib>:"Unset Busy.vi"("error in (no error)"=w219) -> ("error out"=w218:errorcluster)  [unwired: 10 in]
                  }
                  frame "Busy" {
                    n83 = call <vilib>:"Set Busy.vi"("error in (no error)"=w221) -> ("error out"=w220:errorcluster)  [unwired: 9 in, 1 out]
                  }
                }
              }
            }
            n84 = call <vilib>:"Add State(s) to Queue__jki_lib_state_machine.vi"("State(s) in (\"\")"=w213) -> ("States Out"=w212:string)  [unwired: 14 in]
          }
          frame "UI: Front Panel State" {
            # "use for debugging"
            # "Argument"
            # "Set Front Panel Open or Closed\n(Usage: \"UI: Front Panel State >> Open|Close\")"
            n85 = Unbundle By Name(w228) -> ("Core.Current VI Reference"=w227:refnum<vi>)
            n86 = disable-structure shown="Default" {
              disable-tunnel: w229 -> [w235 w258]
              disable-tunnel: [w234 w258] -> w224
              disable-tunnel: w227 -> [w233 _]
              disable-tunnel: w226 -> [w232 _]
              frame condition #0 (active) {
                n87 = case shown="\"Close\"" w232 {
                  tunnel: w235 -> [w239 w252]
                  tunnel: [w241 w253] -> w234
                  tunnel: w233 -> [w240 w250]
                  frame "Open", Default {
                    n88 = property class="VI"(reference=w240, error in=w239) -> (reference out=w237:refnum<vi>, error out=w238:errorcluster, "FP.State"=w236:T15)
                    n89 = case shown="\"Closed\"" w236 {
                      tunnel: [w244 w247] -> w241
                      tunnel: w238 -> [w243 w247]
                      tunnel: w237 -> [w242 _]
                      frame "Closed" {
                        n90 = invoke class="VI" method="FP.Open"(reference=w242, error in=w243, "Activate"=TRUE, "State"=T15."Standard") -> (error out=w244:errorcluster)  [unwired: 1 in, 4 out]
                      }
                      frame Default {
                      }
                    }
                  }
                  frame "Close" {
                    n91 = property class="VI"(reference=w250, error in=w252) -> (reference out=w249:refnum<vi>, error out=w251:errorcluster, "FP.State"=w248:T15)
                    n92 = case shown="Default" w248 {
                      tunnel: [w254 w257] -> w253
                      tunnel: w251 -> [w254 w256]
                      tunnel: w249 -> [_ w255]
                      frame "Invalid", "Closed" {
                      }
                      frame Default {
                        n93 = invoke class="VI" method="FP.Close"(reference=w255, error in=w256) -> (error out=w257:errorcluster)  [unwired: 1 in, 2 out]
                      }
                    }
                  }
                }
              }
              frame condition #1 {
              }
            }
            n94 = call <userlib>:"Wait (ms)__ogtk.vi"("error in (no error)"=w224, "milliseconds to wait"=u32 0) -> ("error out"=w223:errorcluster)  [unwired: 8 in, 1 out]
            n95 = call <vilib>:"Add State(s) to Queue__jki_lib_state_machine.vi"("State(s) in (\"\")"=w231) -> ("States Out"=w230:string)  [unwired: 14 in]
          }
          frame "---------- Macro ----------" {
            # "Do not put any code in this frame.\n(It is a separator no-op. You can make a copy of this frame to create a new Macro frame)"
            n96 = call <vilib>:"Add State(s) to Queue__jki_lib_state_machine.vi"("State(s) in (\"\")"=w263) -> ("States Out"=w262:string)  [unwired: 14 in]
          }
          frame "Macro: Initialize" {
            w264 = "Process: Sync"
            # "Initialization Macro\n(This is called once, when the VI starts)"
            n97 = control-ref of="This VI"() -> (w266:refnum<vi>)
            n98 = property class="VI"(reference=w266) -> ("Exec.State"=w265:T16)  [unwired: 1 in, 2 out]
            n99 = Equal?(x=w265, y=T16."Run top level") -> (x = y?=w271:bool)
            n100 = Select(t=w264, s=w271, f="") -> ()  [unwired: 1 out]
            n101 = call <vilib>:"Add State(s) to Queue__jki_lib_state_machine.vi"("State(s) in Front (\"\")"="Data: Initialize\nInitialize Core Data\nUI: Initialize\nUI: Front Panel State >> Close\nDAQ: update config\nDAQ: init\nEvents: Register", "State(s) in (\"\")"=w264, "State(s) at Back (\"\")"="DAQ: start SMO") -> ("States Out"=w267:string)  [unwired: 12 in]
            n102 = call <vilib>:"Add State(s) to Queue__jki_lib_state_machine.vi"("State(s) in Front (\"\")"=w267, "State(s) in (\"\")"=w277) -> ("States Out"=w276:string)  [unwired: 13 in]
          }
          frame "Macro: Exit" {
            # "Exit Macro\n(This is called once, when the VI exits)"
            n103 = Unbundle By Name(w283) -> ("Core.Close Panel on Exit?"=w289:bool)
            n104 = Select(t="UI: Front Panel State >> Close", s=w289, f="") -> (s? t:f=w286:string)
            n105 = call <vilib>:"Add State(s) to Queue__jki_lib_state_machine.vi"("State(s) in Front (\"\")"="Data: Cleanup\nEvents: Unregister", "State(s) in (\"\")"="Process: Sync", "State(s) at Back (\"\")"="Exit") -> ("States Out"=w280:string)  [unwired: 12 in]
            n106 = call <vilib>:"Add State(s) to Queue__jki_lib_state_machine.vi"("State(s) in Front (\"\")"="DAQ: stop SMO", "State(s) in (\"\")"=w286, "State(s) at Back (\"\")"=w280) -> ("States Out"=w285:string)  [unwired: 12 in]
            n107 = call <vilib>:"Add State(s) to Queue__jki_lib_state_machine.vi"("State(s) in Front (\"\")"=w285, "State(s) in (\"\")"=w292) -> ("States Out"=w291:string)  [unwired: 13 in]
          }
          frame "---------- Process ----------" {
            # "Template Separator\n(You can make a copy of, or modify, this frame)"
            n108 = call <vilib>:"Add State(s) to Queue__jki_lib_state_machine.vi"("State(s) in (\"\")"=w297) -> ("States Out"=w296:string)  [unwired: 14 in]
          }
          frame "Process: Sync" {
            n109 = Unbundle By Name(w305) -> ("Self Reference"=w301:refnum<class "DAQ_Manager.lvclass">)
            n110 = call <vilib>:"WaitOnProcessSync.vi"("error in (no error)"=w300, "SMO"=w301) -> ("error out"=w299:errorcluster, "Don't run?"=w304:bool)  [unwired: 7 in, 1 out]
            n111 = Select(t="Data: Cleanup\nEvents: Unregister\nExit", s=w304, f="") -> (s? t:f=w298:string)
            n112 = call <vilib>:"Add State(s) to Queue__jki_lib_state_machine.vi"("State(s) in Front (\"\")"=w298, "State(s) in (\"\")"=w308) -> ("States Out"=w307:string)  [unwired: 13 in]
          }
          frame "---------- Events ----------" {
            # "Template Separator\n(You can make a copy of, or modify, this frame)"
            n113 = call <vilib>:"Add State(s) to Queue__jki_lib_state_machine.vi"("State(s) in (\"\")"=w313) -> ("States Out"=w312:string)  [unwired: 14 in]
          }
          frame "Events: Register" {
            # "GetPublicEvents of DAQManager"
            # "GetPublicEvents of DAQ"
            # "GetPrivateEvents of DAQManager"
            n114 = Unbundle By Name(w323) -> ("Self Reference"=w329:refnum<class "DAQ_Manager.lvclass">)
            n115 = call <vilib>:"GetProtectedEvents.vi"("error in (no error)"=w327, "SMO"=w329) -> ("error out"=w320:errorcluster, "SMO Protected Events"=w325:T22, "SMO out"=w321:refnum<class "DAQ_Manager.lvclass">)  [unwired: 7 in]
            n116 = Unbundle By Name(w323) -> ("DAQ"=w315:refnum<class "DAQ.lvclass">[])
            n117 = call "DAQ_Manager.GetPrivateEvents.vi"("error in (no error)"=w320, "DAQ_Manager"=w321) -> ("error out"=w317:errorcluster, "Private Events"=w326:T23, "DAQ_Manager out"=w318:refnum<class "DAQ_Manager.lvclass">)  [unwired: 7 in]
            n118 = call "DAQ_Manager.GetPublicEvents.vi"("error in (no error)"=w317, "DAQ_Manager"=w318) -> ("error out"=w316:errorcluster, "Public Events"=w319:T24)  [unwired: 7 in, 1 out]
            n119 = for {
              tunnel: w315 -> [w337] mode=indexing
              shift-right: [w335] -> _
              shift-left: w316 -> [w336]
              tunnel: [w333] -> w324 mode=indexing
              n120 = call "DAQ.GetPublicEvents.vi"("error in (no error)"=w336, "DAQ"=w337) -> ("error out"=w335:errorcluster, "Public Events"=w334:T25)  [unwired: 7 in, 1 out]
              n121 = Unbundle By Name(w334) -> ("DAQ.Read"=w333:refnum<user-event>)
            }
            n122 = call "RenameReadEvents.vi"("DAQ.Read"=w324) -> ("DAQ.Read"=w314:refnum<user-event>[])
            n123 = register-events(w325, w326, w319, w314) -> (reference out=w330:refnum<event-registration>, error out=w328:errorcluster)  [unwired: 2 in]
            n124 = Bundle By Name(cluster=w323, "AI events"=w314) -> (w322:T18)
            n125 = call <vilib>:"Add State(s) to Queue__jki_lib_state_machine.vi"("State(s) in (\"\")"=w332) -> ("States Out"=w331:string)  [unwired: 14 in]
          }
          frame "Events: Unregister" {
            n126 = Unregister For Events(event registration refnum=w340, error in=w339) -> (error out=w338:errorcluster)
            n127 = call <vilib>:"Clear Errors.vi"("error in (no error)"=w338) -> ()  [unwired: 5 in, 2 out]
            n128 = call <vilib>:"Add State(s) to Queue__jki_lib_state_machine.vi"("State(s) in (\"\")"=w343) -> ("States Out"=w342:string)  [unwired: 14 in]
          }
          frame "---------- DAQ ----------" {
            n129 = call <vilib>:"Add State(s) to Queue__jki_lib_state_machine.vi"("State(s) in (\"\")"=w348) -> ("States Out"=w347:string)  [unwired: 14 in]
          }
          frame "DAQ: init" {
            # "I don't think TO is relevant here. More important for DAQ SMO?"
            n130 = Unbundle By Name(w352) -> ("DAQ.Config (AI)"=w358:T7[], "DAQmx.AI.Config"=w355:T4[], "DAQ.Config (AO)"=w357:T7[], "DAQmx.AO.Config"=w356:T2[])
            n131 = case shown="False" "Simulate?" {
              tunnel: w357 -> [w376 w395]
              tunnel: w356 -> [w375 _]
              tunnel: w358 -> [w374 w394]
              tunnel: w355 -> [w373 _]
              tunnel: [w368 w388] -> w354
              tunnel: [w367 w389] -> w350
              tunnel: w353 -> [w364 w387]
              frame False {
                n132 = for {
                  tunnel: w376 -> [w381] mode=indexing
                  tunnel: w375 -> [w380] mode=indexing
                  tunnel: [w379] -> w371 mode=indexing
                  shift-right: [w378] -> w369
                  shift-left: w364 -> [w377]
                  n133 = call "createDAQmx.AO.vi"("error in (no error)"=w377, "DAQmx.AO.config"=w380, "DAQ.Config"=w381) -> ("error out"=w378:errorcluster, "DAQmx.AO out"=w379:refnum<class "DAQmx.AO.lvclass">)  [unwired: 7 in]
                }
                n134 = for {
                  tunnel: w374 -> [w386] mode=indexing
                  tunnel: w373 -> [w385] mode=indexing
                  tunnel: [w383] -> w372 mode=indexing
                  shift-right: [w384] -> w370
                  shift-left: w364 -> [w382]
                  n135 = call "createDAQmx.AI.vi"("error in (no error)"=w382, "DAQmx.AI.config"=w385, "DAQ.config"=w386) -> ("error out"=w384:errorcluster, "DAQmx.AI out"=w383:refnum<class "DAQmx.AI.lvclass">)  [unwired: 7 in]
                }
                n136 = Merge Errors(w370, w369) -> (w365:errorcluster)
                n137 = Build Array (concatenate)(w372, w371) -> (w366:refnum<class "DAQmx.lvclass">[])
                n138 = call "DAQmx_SyncAll.vi"("error in (no error)"=w365, "Array in"=w366) -> ("error out"=w368:errorcluster, "Array out"=w367:refnum<class "DAQmx.lvclass">[])  [unwired: 8 in]
              }
              frame True {
                n139 = for {
                  tunnel: w394 -> [w403] mode=indexing
                  tunnel: [w402] -> w393 mode=indexing
                  shift-right: [w401] -> w391
                  shift-left: w387 -> [w400]
                  n140 = call "createDAQ.vi"("error in (no error)"=w400, "DAQ.Config"=w403) -> ("error out"=w401:errorcluster, "DAQ out"=w402:refnum<class "DAQ.lvclass">)  [unwired: 8 in]
                }
                n141 = for {
                  tunnel: w395 -> [w399] mode=indexing
                  tunnel: [w398] -> w392 mode=indexing
                  shift-right: [w397] -> w390
                  shift-left: w387 -> [w396]
                  n142 = call "createDAQ.vi"("error in (no error)"=w396, "DAQ.Config"=w399) -> ("error out"=w397:errorcluster, "DAQ out"=w398:refnum<class "DAQ.lvclass">)  [unwired: 8 in]
                }
                n143 = Build Array (concatenate)(w393, w392) -> (w389:refnum<class "DAQ.lvclass">[])
                n144 = Merge Errors(w391, w390) -> (w388:errorcluster)
              }
            }
            n145 = Unbundle By Name(w352) -> ("Self Reference"=w351:refnum<class "DAQ_Manager.lvclass">)
            n146 = Bundle By Name(cluster=w351, "DAQ"=w350) -> (w349:refnum<class "DAQ_Manager.lvclass">)
            n147 = Bundle By Name(cluster=w352, "Self Reference"=w349, "DAQ"=w350) -> (w360:T18)
            n148 = call <vilib>:"Add State(s) to Queue__jki_lib_state_machine.vi"("State(s) in (\"\")"=w363) -> ("States Out"=w362:string)  [unwired: 14 in]
          }
          frame "DAQ: start SMO" {
            n149 = Unbundle By Name(w404) -> ("Self Reference"=w405:refnum<class "DAQ_Manager.lvclass">)
            n150 = Unbundle By Name(w404) -> ("DAQ"=w406:refnum<class "DAQ.lvclass">[])
            n151 = for {
              shift-right: [w412] -> w407
              shift-left: w408 -> [w413]
              tunnel: w406 -> [w414] mode=indexing
              tunnel: w405 -> [_]
              n152 = call <vilib>:"Start.vi"("error in (no error)"=w413, "SMO"=w414) -> ("error out"=w412:errorcluster)  [unwired: 8 in, 1 out]
            }
            n153 = call <vilib>:"Add State(s) to Queue__jki_lib_state_machine.vi"("State(s) in (\"\")"=w411) -> ("States Out"=w410:string)  [unwired: 14 in]
          }
          frame "DAQ: stop SMO" {
            n154 = Unbundle By Name(w420) -> ("DAQ"=w415:refnum<class "DAQ.lvclass">[])
            n155 = for {
              tunnel: w415 -> [w428] mode=indexing
              tunnel: w419 -> [w429]
              tunnel: [w425] -> w418 mode=indexing
              tunnel: [w424] -> w416 mode=indexing
              n156 = call <vilib>:"Stop.vi"("error in (no error)"=w429, "SMO"=w428) -> ("error out"=w427:errorcluster, "SMO out"=w426:refnum<class "DAQ.lvclass">)  [unwired: 8 in]
              n157 = call <vilib>:"GetState.vi"("error in (no error)"=w427, "SMO"=w426) -> ("error out"=w425:errorcluster, "SMO State"=w424:T1)  [unwired: 7 in, 1 out]
            }
            "Array" <- w416
            n158 = Merge Errors(w418) -> (w417:errorcluster)
            n159 = call <vilib>:"Add State(s) to Queue__jki_lib_state_machine.vi"("State(s) in (\"\")"=w423) -> ("States Out"=w422:string)  [unwired: 14 in]
          }
          frame "DAQ: destroy SMO" {
            n160 = Unbundle By Name(w434) -> ("DAQ"=w430:refnum<class "DAQ.lvclass">[])
            n161 = for {
              tunnel: w430 -> [w439] mode=indexing
              tunnel: w433 -> [w440]
              tunnel: [w438] -> w432 mode=indexing
              n162 = call <vilib>:"Destroy.vi"("error in (no error)"=w440, "SMO"=w439) -> ("error out"=w438:errorcluster)  [unwired: 9 in]
            }
            n163 = Merge Errors(w432) -> (w431:errorcluster)
            n164 = call <vilib>:"Add State(s) to Queue__jki_lib_state_machine.vi"("State(s) in (\"\")"=w437) -> ("States Out"=w436:string)  [unwired: 14 in]
          }
          frame "DAQ: update config" {
            n165 = Bundle By Name(cluster=w442, "DAQ.Config (AO)"="DAQ.Config (AO)", "DAQ.Config (AI)"="DAQ.Config (AI)", "DAQmx.AO.Config"="DAQmx.AO.config", "DAQmx.AI.Config"="DAQmx.AI.config") -> (w441:T18)
            n166 = call <vilib>:"Add State(s) to Queue__jki_lib_state_machine.vi"("State(s) in (\"\")"=w449) -> ("States Out"=w448:string)  [unwired: 14 in]
          }
          frame "DAQ: setWaveform" {
            # "concatenate channels and send to DAQ SMOs"
            # "figure out which are AO channels"
            n167 = Unbundle By Name(w457) -> ("DAQ"=w451:refnum<class "DAQ.lvclass">[], "setWaveform"=w452:T17)
            n168 = call "DAQ_Manager.getAO_chan_and_sampling.vi"("error in (no error)"=w453, "DAQ"=w451) -> ("error out"=w455:errorcluster, "DAQ (AO)"=w456:refnum<class "DAQ.lvclass">[])  [unwired: 6 in, 2 out]
            n169 = call "Concatenate_and_SetWaveforms.vi"("error in (no error)"=w455, "AO Array"=w452, "DAQ (AO)"=w456) -> ("error out"=w454:errorcluster)  [unwired: 6 in, 2 out]
            n170 = call <vilib>:"Add State(s) to Queue__jki_lib_state_machine.vi"("State(s) in (\"\")"=w460) -> ("States Out"=w459:string)  [unwired: 14 in]
          }
        }
      }
    }
    frame Error {
    }
  }
  n171 = call-parent "Process.vi"("error in"=w9, "SMO"=w8) -> ("error out"=w6:errorcluster, "SMO out"=→"DAQ_Manager out":refnum<class "DAQ_Manager.lvclass">)  [unwired: 8 in]
  n172 = Merge Errors(w6, w5) -> (→"error out":errorcluster)
